vi "dual_gate_absorption.vi"() -> ()   [LabVIEW 2010]
uses:
  <vilib>/Utility/file.llb/Write To Spreadsheet File (DBL).vi
  <instrlib>/lib-labview-8.6-export/Keithley-6482-Visa.lvlib
panel:
  out "Error Out":errorcluster
  in  "Error In":errorcluster
  out "Current V2":dbl
  out "V2 delta":dbl
  in  "V2 end":dbl=-2.0
  in  "V2 start":dbl=2.0
  in  "V2 step":dbl=0.1
  out "V1 delta":dbl
  in  "V1 end":dbl=-2.0
  in  "V1 start":dbl=2.0
  in  "V1 step":dbl=0.1
  in  "base path":path=path "C:/Users/Pump probe_B145/Desktop/data/2019/190630/gate_abs/GBG_N1V_GBG_2VtoN2V_GBGregion"
  in  "xoffset":u16=1
  in  "width":u16=1340
  in  "xbin":u16=1
  in  "Integrations":i32=1
  in  "yoffset":u16=1
  in  "height":u16=100
  in  "ybin":u16=1
  in  "Center wavelength":dbl=650.0
  in  "Grating":bool=TRUE
  in  "Exposure time (s)":dbl=0.1 format="%.2f"
  out "XY Graph":cluster{dbl[], dbl[]}(graph) caption="Spectrum"
  in  "File name":string="HT78_300G_650C_0.1s_100int_15swait"
  in  "initial wait (ms)":dbl=300000.0
  in  "wait time (ms)`":dbl=15000.0
  out "Current V1":dbl
  out "Current":dbl[](array[numeric])
  in  "VISA resource name":refnum<visa-resource-name>="GPIB0::20::INSTR"
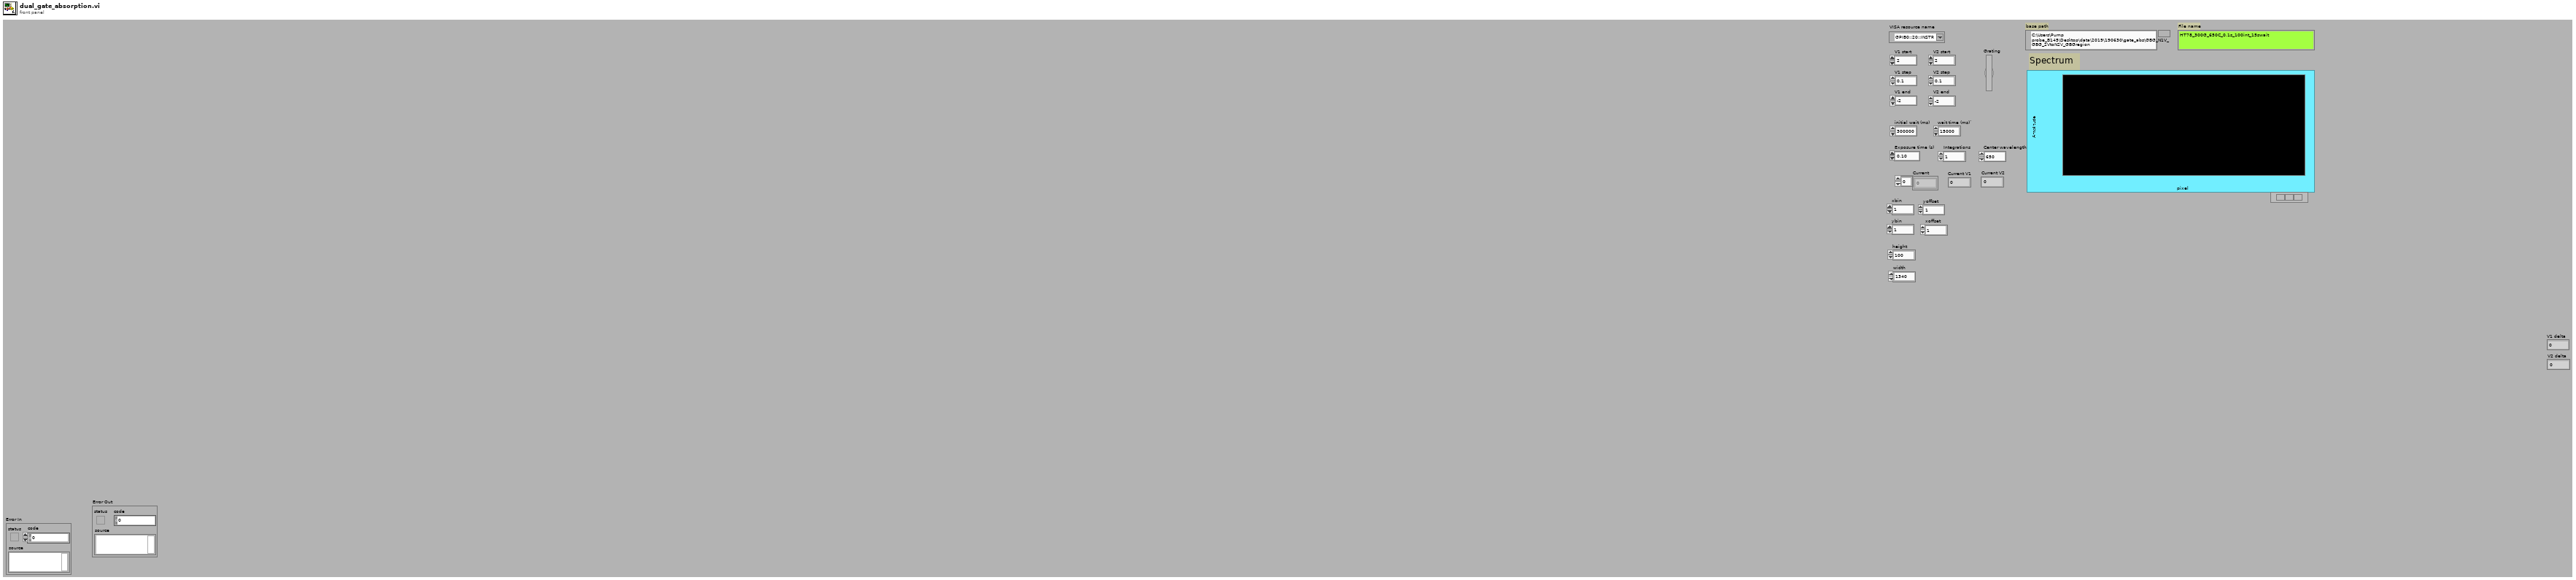
[diagram p1: front panel]
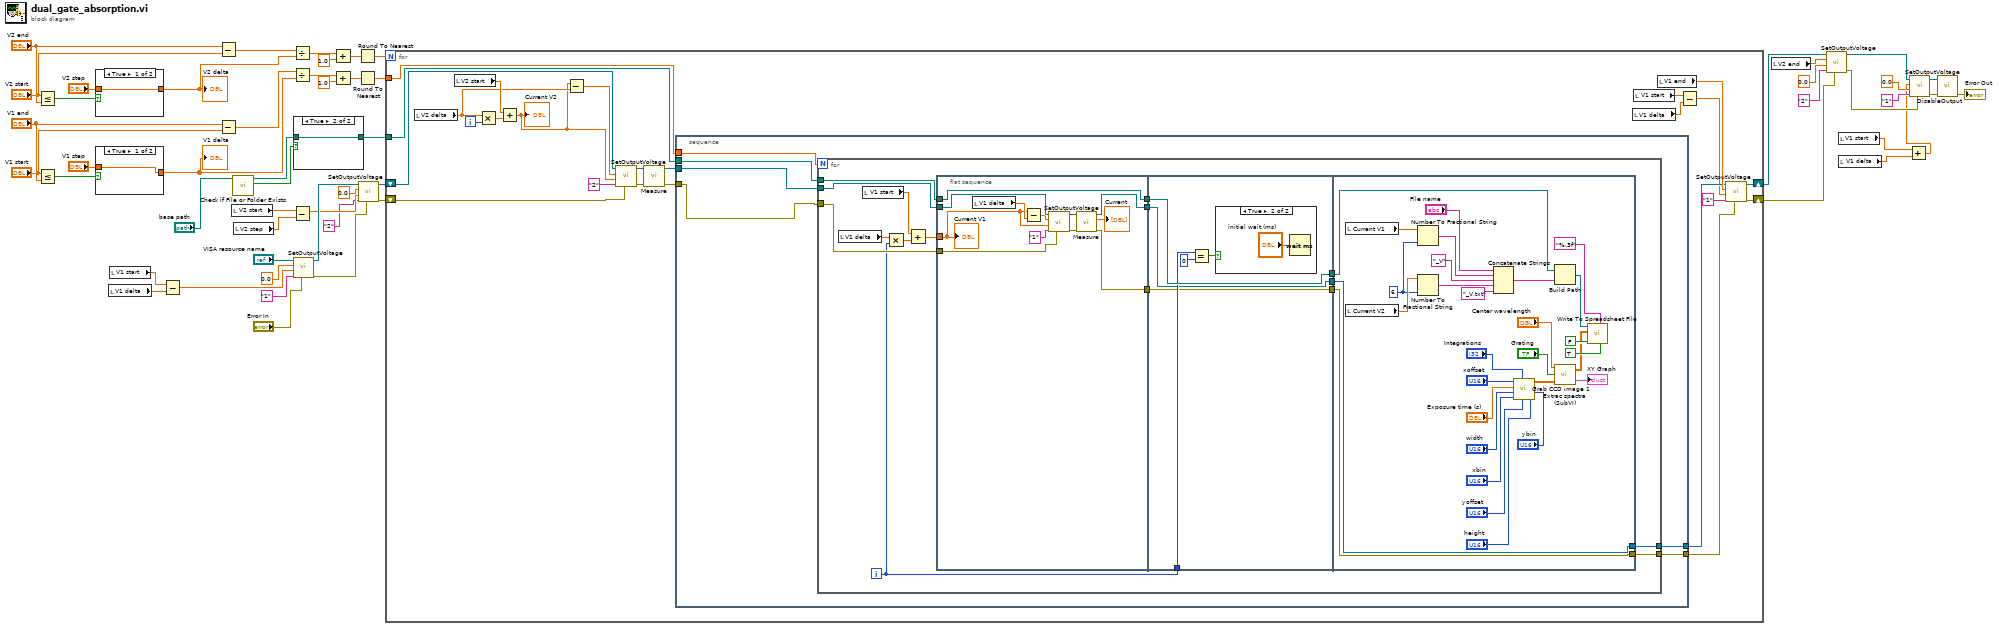
[diagram p0: block diagram]
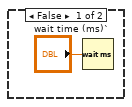
[diagram p2: hidden frame]
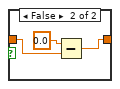
[diagram p3: hidden frame]
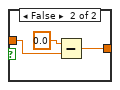
[diagram p4: hidden frame]
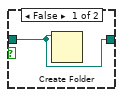
[diagram p5: hidden frame]
diagram:
  n1 = Less Or Equal?(x="V2 start", y="V2 end") -> (x <= y?=w41:bool)
  n2 = Less Or Equal?(x="V1 start", y="V1 end") -> (x <= y?=w51:bool)
  n3 = case shown="True" w41 {
    tunnel: "V2 step" -> [w56 w58]
    tunnel: [w56 w57] -> w36
    frame True {
    }
    frame False {
      n4 = Subtract(x=0.0, y=w58) -> (x-y=w57:dbl)
    }
  }
  "V2 delta" <- w36
  n5 = case shown="True" w51 {
    tunnel: "V1 step" -> [w60 w62]
    tunnel: [w60 w61] -> w46
    frame True {
    }
    frame False {
      n6 = Subtract(x=0.0, y=w62) -> (x-y=w61:dbl)
    }
  }
  "V1 delta" <- w46
  n7 = local read "V1 delta"() -> (w23:dbl)
  n8 = local read "V1 start"() -> (w24:dbl)
  n9 = Subtract(x=w24, y=w23) -> (x-y=w22:dbl)
  n10 = Subtract(x="V2 end", y="V2 start") -> (x-y=w37:dbl)
  n11 = Subtract(x="V1 end", y="V1 start") -> (x-y=w47:dbl)
  n12 = local read "V2 start"() -> (w13:dbl)
  n13 = call <vilib>:"Check if File or Folder Exists.vi"("path"="base path") -> ("file or folder exists?"=w54:bool, "dup path"=w55:path)  [unwired: 8 in, 1 out]
  n14 = local read "V2 step"() -> (w12:dbl)
  n15 = Divide(x=w37, y=w36) -> (x/y=w35:dbl)
  n16 = Divide(x=w47, y=w46) -> (x/y=w45:dbl)
  n17 = Subtract(x=w13, y=w12) -> (x-y=w11:dbl)
  n18 = case shown="True" w54 {
    tunnel: w55 -> [w64 w65]
    tunnel: [w64 w65] -> w52
    frame False {
      n19 = Create Folder(path (use dialog)=w64) -> ()  [unwired: 2 in, 3 out]
    }
    frame True {
    }
  }
  n20 = call <instrlib>:"SetOutputVoltage.vi"("Error In"="Error In", "channel(1,2)"="1", "Voltage"=w22, "V_pre"=0.0, "Keithley 6482"="VISA resource name") -> ("Error Out"=w18:errorcluster, "Keithley 6483"=w15:refnum<visa-resource-name>)  [unwired: 5 in]
  n21 = Add(x=w35, y=1.0) -> (x+y=w33:dbl)
  n22 = Add(x=w45, y=1.0) -> (x+y=w43:dbl)
  n23 = Round To Nearest(number=w33) -> (nearest integer value=w32:dbl)
  n24 = Round To Nearest(number=w43) -> (nearest integer value=w42:dbl)
  n25 = call <instrlib>:"SetOutputVoltage.vi"("Error In"=w18, "channel(1,2)"="2", "Voltage"=w11, "V_pre"=0.0, "Keithley 6482"=w15) -> ("Error Out"=w17:errorcluster, "Keithley 6483"=w16:refnum<visa-resource-name>)  [unwired: 5 in]
  n26 = for {
    N: w32 -> [_]
    tunnel: w52 -> [w89]
    tunnel: w42 -> [w88]
    shift-right: [w83] -> w27
    shift-left: w16 -> [w70]
    shift-right: [w82] -> w29
    shift-left: w17 -> [w69]
    i -> [w78]
    n27 = local read "V2 delta"() -> (w75:dbl)
    n28 = local read "V2 start"() -> (w77:dbl)
    n29 = Multiply(x=w75, y=w78) -> (x*y=w76:dbl)
    n30 = Add(x=w77, y=w76) -> (x+y=w73:dbl)
    "Current V2" <- w73
    n31 = Subtract(x=w73, y=w75) -> (x-y=w74:dbl)
    n32 = call <instrlib>:"SetOutputVoltage.vi"("Error In"=w69, "channel(1,2)"="2", "Voltage"=w73, "V_pre"=w74, "Keithley 6482"=w70) -> ("Error Out"=w80:errorcluster, "Keithley 6483"=w81:refnum<visa-resource-name>)  [unwired: 5 in]
    n33 = call <instrlib>:"Measure.vi"("Error In"=w80, "Keithley 6482 In"=w81) -> ("Error Out"=w71:errorcluster, "Keithley 6482 Out"=w72:refnum<visa-resource-name>)  [unwired: 7 in, 1 out]
    n34 = stacked-sequence {
      tunnel: w72 -> [w91]
      tunnel: w89 -> [w95]
      tunnel: [w94] -> w85
      tunnel: [w93] -> w84
      tunnel: w88 -> [w92]
      tunnel: w71 -> [w90]
      frame #0 {
        n35 = for {
          N: w92 -> [_]
          tunnel: w91 -> [w111]
          tunnel: w95 -> [w110]
          tunnel: [w105] -> w94
          tunnel: [w103] -> w93
          tunnel: w90 -> [w101]
          i -> [w98]
          n36 = local read "V1 delta"() -> (w97:dbl)
          n37 = local read "V1 start"() -> (w100:dbl)
          n38 = Multiply(x=w97, y=w98) -> (x*y=w96:dbl)
          n39 = Add(x=w100, y=w96) -> (x+y=w99:dbl)
          n40 = flat-sequence {
            tunnel: w111 -> [w122]
            tunnel: w99 -> [w113]
            tunnel: [w123] -> w109
            tunnel: w110 -> [w123]
            tunnel: [w119] -> w106
            tunnel: [w117] -> w102
            tunnel: w101 -> [w121]
            tunnel: w109 -> [w129]
            tunnel: [w129] -> w108
            tunnel: w98 -> [w128]
            tunnel: [w125] -> w107
            tunnel: w106 -> [w125]
            tunnel: [w124] -> w104
            tunnel: w102 -> [w124]
            tunnel: w108 -> [w141]
            tunnel: w107 -> [w140]
            tunnel: [w140] -> w105
            tunnel: w104 -> [w139]
            tunnel: [w139] -> w103
            frame #0 {
              n41 = local read "V1 delta"() -> (w114:dbl)
              n42 = Subtract(x=w113, y=w114) -> (x-y=w112:dbl)
              n43 = call <instrlib>:"SetOutputVoltage.vi"("Error In"=w121, "channel(1,2)"="1", "Voltage"=w113, "V_pre"=w112, "Keithley 6482"=w122) -> ("Error Out"=w118:errorcluster, "Keithley 6483"=w120:refnum<visa-resource-name>)  [unwired: 5 in]
              n44 = call <instrlib>:"Measure.vi"("Error In"=w118, "Keithley 6482 In"=w120) -> ("Error Out"=w117:errorcluster, "Values"=→"Current":dbl[], "Keithley 6482 Out"=w119:refnum<visa-resource-name>)  [unwired: 7 in]
              "Current V1" <- w113
            }
            frame #1 {
              n45 = Equal?(x=w128, y=0) -> (x = y?=w127:bool)
              n46 = case shown="True" w127 {
                frame False {
                  n47 = Wait (ms)(milliseconds to wait="wait time (ms)`") -> ()  [unwired: 1 out]
                }
                frame True {
                  n48 = Wait (ms)(milliseconds to wait="initial wait (ms)") -> ()  [unwired: 1 out]
                }
              }
            }
            frame #2 {
              w135 = 6
              n49 = local read "Current V1"() -> (w137:dbl)
              n50 = local read "Current V2"() -> (w136:dbl)
              n51 = Number To Fractional String(number=w137, precision (6)=w135) -> (F-format string=w133:string)  [unwired: 2 in]
              n52 = Number To Fractional String(number=w136, precision (6)=w135) -> (F-format string=w134:string)  [unwired: 2 in]
              n53 = Concatenate Strings("File name", w133, "_V" ("string"), w134, "_V.txt" ("Substring")) -> (w143:string)
              n54 = call "Grab CCD image 1.vi"("height"="height", "ybin"="ybin", "yoffset"="yoffset", "Average time"="Integrations", "xbin"="xbin", "width"="width", "Exposure time (s)"="Exposure time (s)", "xoffset"="xoffset") -> ("CCD image"=w152:dbl[][])  [unwired: 1 out]
              n55 = Build Path(base path=w141, name or relative path=w143) -> (appended path=w142:path)
              n56 = call "Extrac spectra (SubVI).vi"("CCD image"=w152, "Grating (1:300nm/0:1200nm)"="Grating", "Center wavelength"="Center wavelength") -> ("XY Graph"=→"XY Graph":cluster{dbl[], dbl[]}, "appended array"=w145:dbl[][])
              n57 = call-poly <vilib>:"Write To Spreadsheet File.vi"("transpose? (no:F)"=TRUE, "format (%.3f)"="%.3f", "append to file? (new file:F)"=FALSE, "2D data"=w145, "file path (dialog if empty)"=w142) -> ()  [unwired: 3 in, 1 out]
            }
          }
        }
      }
    }
    n58 = local read "V1 delta"() -> (w67:dbl)
    n59 = local read "V1 start"() -> (w68:dbl)
    n60 = local read "V1 end"() -> (w86:dbl)
    n61 = Subtract(x=w68, y=w67) -> (x-y=w66:dbl)
    n62 = call <instrlib>:"SetOutputVoltage.vi"("Error In"=w84, "channel(1,2)"="1", "Voltage"=w66, "V_pre"=w86, "Keithley 6482"=w85) -> ("Error Out"=w82:errorcluster, "Keithley 6483"=w83:refnum<visa-resource-name>)  [unwired: 5 in]
  }
  n63 = local read "V2 end"() -> (w26:dbl)
  n64 = call <instrlib>:"SetOutputVoltage.vi"("Error In"=w29, "channel(1,2)"="2", "Voltage"=0.0, "V_pre"=w26, "Keithley 6482"=w27) -> ("Error Out"=w5:errorcluster, "Keithley 6483"=w9:refnum<visa-resource-name>)  [unwired: 5 in]
  n65 = local read "V1 start"() -> (w3:dbl)
  n66 = local read "V1 delta"() -> (w2:dbl)
  n67 = Add(x=w3, y=w2) -> (x+y=w1:dbl)
  n68 = call <instrlib>:"SetOutputVoltage.vi"("Error In"=w5, "channel(1,2)"="1", "Voltage"=0.0, "V_pre"=w1, "Keithley 6482"=w9) -> ("Error Out"=w7:errorcluster, "Keithley 6483"=w8:refnum<visa-resource-name>)  [unwired: 5 in]
  n69 = call <instrlib>:"DisableOutput.vi"("Error In"=w7, "Keithley 6482 In"=w8) -> ("Error Out"=→"Error Out":errorcluster)  [unwired: 8 in, 1 out]
